vi "Handle Messages.vi"(8 "error in (no error)":errorcluster, 9 "Message Data":variant, 10 "Message":string, 11 "Process In":refnum<class "Process.lvclass">) -> (0 "error out":errorcluster, 3 "Process Out":refnum<class "Process.lvclass">)   [LabVIEW 2020, in "Process.lvclass"]
doc: "This is the core VI handling incomming messages to the process. This VI should be overridden to add functionality to the process or override functionality implemented by a parent. Any message not handled should be sent to the parent method using the default case. \nEach state should be atomic and states should in general avoid enqueueing new messages from within this method, as there might be other messages interleaved in the queue from the outside. For cyclic iteration of an action, using a Helper Loop is recommended."
uses:
  Process.lvclass
  C:/Users/anton/Documents/GitHub/Triarc-Framework/source/Framework/Logging/Logging.lvclass
  C:/Users/anton/Documents/GitHub/Triarc-Framework/source/Framework/Base/Base.lvclass
  Public/Lifecycle/Lifecycle State.ctl
  Process.lvclass/Process.ctl
  Error Handler Interface/Error Handler Interface.lvclass
  Logging/Logging.lvclass
  Public/Lifecycle/Leave Process Loop.vi
  <vilib>/Utility/error.llb/Clear Errors.vi
  <vilib>/Utility/error.llb/Error Cluster From Error Code.vi
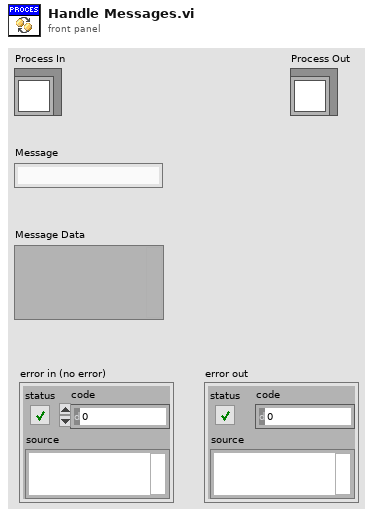
[diagram p1: front panel]
types:
  T1 = typedef "Process.lvclass/Lifecycle State.ctl" = enum16{"Uninitialized", "Initialized", "Started", "Running", "Stopped", "Finished"}
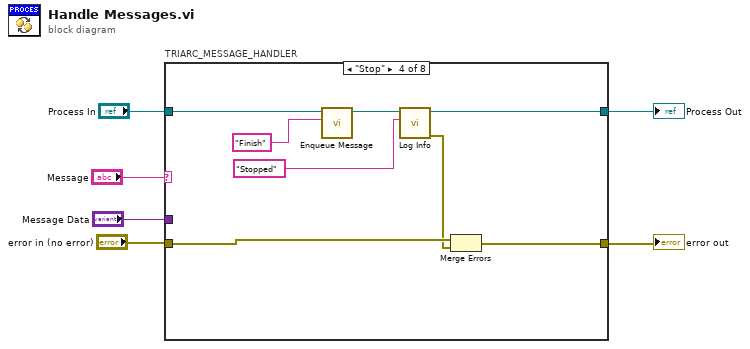
[diagram p0: block diagram]
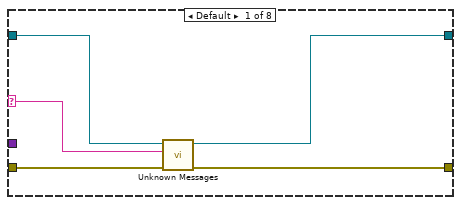
[diagram p2: hidden frame]
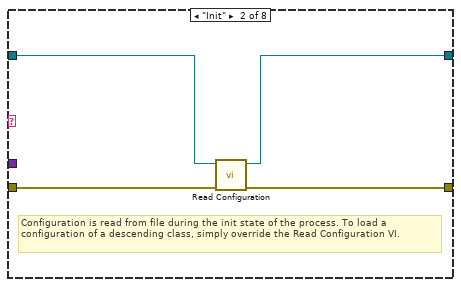
[diagram p3: hidden frame]
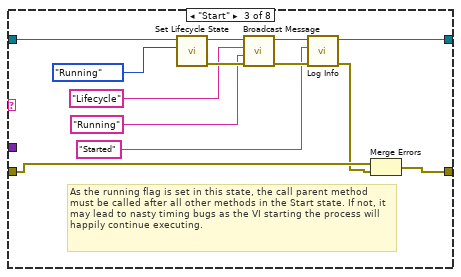
[diagram p4: hidden frame]
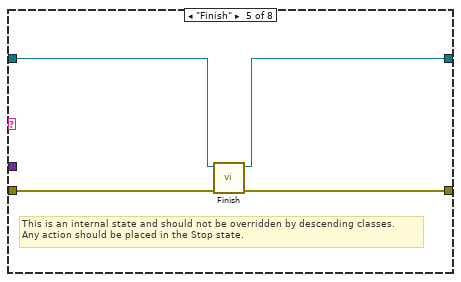
[diagram p5: hidden frame]
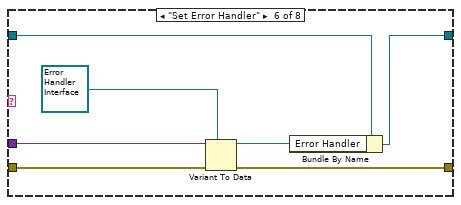
[diagram p6: hidden frame]
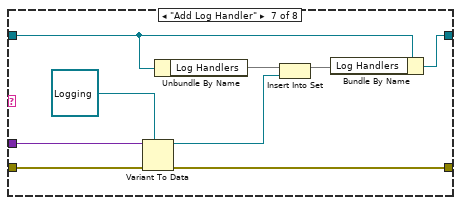
[diagram p7: hidden frame]
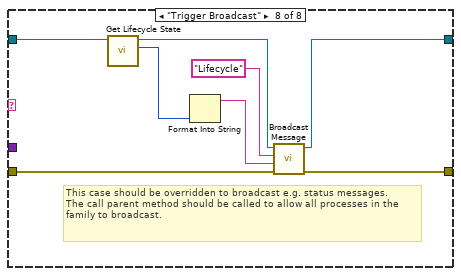
[diagram p8: hidden frame]
diagram:
  n1 = case "TRIARC_MESSAGE_HANDLER" shown="\"Stop\"" "Message" {
    selector: "Message" -> [w11 _ _ _ _ _ _ _]
    tunnel: [w8 w13 w27 w34 w40 w43 w51 w60] -> w5
    tunnel: "error in (no error)" -> [w7 w12 w26 w33 w39 w47 w56 w57]
    tunnel: [w10 w15 w18 w30 w37 w44 w53 w64] -> w3
    tunnel: "Process In" -> [w9 w14 w28 w35 w38 w45 w52 w63]
    tunnel: "Message Data" -> [_ _ _ _ _ w41 w48 _]
    frame Default {
      n2 = call "Unknown Messages.vi"("error in (no error)"=w7, "Message"=w11, "Process In"=w9) -> ("error out"=w8:errorcluster, "Process Out"=w10:refnum<class "Process.lvclass">)  [unwired: 7 in]
    }
    frame "Init" {
      # "Configuration is read from file during the init state of the process. To load a configuration of a descending class, simply override the Read Configuration VI."
      n3 = call-dynamic "Read Configuration.vi"("error in (no error)"=w12, "Process In"=w14) -> ("error out"=w13:errorcluster, "Process Out"=w15:refnum<class "Process.lvclass">)  [unwired: 8 in]
    }
    frame "Start" {
      # "As the running flag is set in this state, the call parent method must be called after all other methods in the Start state. If not, it may lead to nasty timing bugs as the VI starting the process will happily continue executing."
      n4 = call "Set Lifecycle State.vi"("Lifecycle State"=Lifecycle_State."Running", "Process In"=w28) -> ("error out"=w24:errorcluster, "Process Out"=w25:refnum<class "Process.lvclass">)  [unwired: 8 in]
      n5 = call-dynamic "Broadcast Message.vi"("error in (no error)"=w24, "Message Data"="Running" ("Message"), "Message"="Lifecycle", "Rig Process In"=w25) -> ("error out"=w23:errorcluster, "Rig Process Out"=w19:refnum<class "Process.lvclass">)  [unwired: 6 in]
      n6 = call "Log Info.vi"("error in (no error)"=w23, "Message"="Started", "Logging In"=w19) -> ("error out"=w20:errorcluster, "Logging Out"=w18:refnum<class "Process.lvclass">)  [unwired: 7 in]
      n7 = Merge Errors(w26, w20) -> (w27:errorcluster)
    }
    frame "Stop" {
      n8 = call "Enqueue Message.vi"("Message"="Finish", "Process In"=w35) -> ("Process Out"=w31:refnum<class "Process.lvclass">)  [unwired: 8 in, 1 out]
      n9 = call "Log Info.vi"("Message"="Stopped", "Logging In"=w31) -> ("error out"=w32:errorcluster, "Logging Out"=w30:refnum<class "Process.lvclass">)  [unwired: 8 in]
      n10 = Merge Errors(w33, w32) -> (w34:errorcluster)
    }
    frame "Finish" {
      # "This is an internal state and should not be overridden by descending classes.\nAny action should be placed in the Stop state."
      n11 = call "Finish.vi"("error in (no error)"=w39, "Process In"=w38) -> ("error out"=w40:errorcluster, "Process Out"=w37:refnum<class "Process.lvclass">)  [unwired: 8 in]
    }
    frame "Set Error Handler" {
      n12 = Variant To Data(error in=w47, type=refnum<class "Error Handler Interface.lvclass"> refnum ("Error Handler Interface.lvclass"), Variant=w41) -> (data=w42:refnum<class "Error Handler Interface.lvclass">, error out=w43:errorcluster)
      n13 = Bundle By Name(cluster=w45, "Error Handler"=w42) -> (w44:refnum<class "Process.lvclass">)
    }
    frame "Add Log Handler" {
      n14 = Variant To Data(error in=w56, type=refnum<class "Logging.lvclass"> refnum ("element"), Variant=w48) -> (data=w49:refnum<class "Logging.lvclass">, error out=w51:errorcluster)
      n15 = Unbundle By Name(w52) -> ("Log Handlers"=w54:set{refnum<class "Logging.lvclass">})
      n16 = Insert Into Set(10:w49, 11:w54) -> (3:w55:set{refnum<class "Logging.lvclass">})  [unwired: 1 out]
      n17 = Bundle By Name(cluster=w52, "Log Handlers"=w55) -> (w53:refnum<class "Process.lvclass">)
    }
    frame "Trigger Broadcast" {
      # "This case should be overridden to broadcast e.g. status messages.\nThe call parent method should be called to allow all processes in the family to broadcast."
      n18 = call "Get Lifecycle State.vi"("Process In"=w63) -> ("Lifecycle State"=w59:T1, "Process Out"=w61:refnum<class "Process.lvclass">)  [unwired: 7 in, 2 out]
      n19 = Format Into String(w59) -> (resulting string=w58:string)  [unwired: 3 in, 1 out]
      n20 = call-dynamic "Broadcast Message.vi"("error in (no error)"=w57, "Message Data"=w58, "Message"="Lifecycle", "Rig Process In"=w61) -> ("error out"=w60:errorcluster, "Rig Process Out"=w64:refnum<class "Process.lvclass">)  [unwired: 6 in]
    }
  }
  "error out" <- w5
  "Process Out" <- w3
